vi "Display Error.vi"(8 "error in (no error)":errorcluster, 10 "Error message":string, 11 "Monitor-Pulse in":refnum<class "Monitor-Pulse.lvclass">) -> (0 "error out":errorcluster, 3 "Monitor-Pulse out":refnum<class "Monitor-Pulse.lvclass">)   [LabVIEW 2016, in "Monitor-Pulse.lvclass"]
uses:
  Monitor-Pulse.lvclass
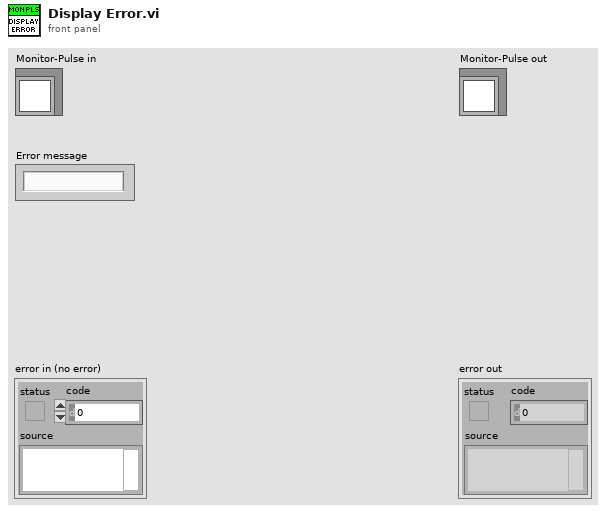
[diagram p1: front panel]
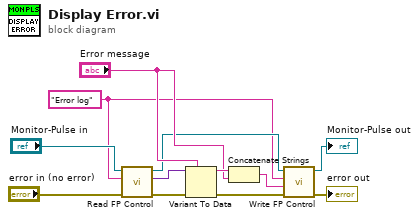
[diagram p0: block diagram]
diagram:
  w6 = "Error log" ("Control Name")
  n1 = call-dynamic "Read FP Control.vi"("error in (no error)"="error in (no error)", "Control Name"=w6, "Measure Object in"="Monitor-Pulse in") -> ("error out"=w10:errorcluster, "Control Value"=w11:variant, "Measure Object out"=w7:refnum<class "Monitor-Pulse.lvclass">)  [unwired: 5 in, 1 out]
  n2 = Variant To Data(error in=w10, type="Error message", Variant=w11) -> (data=w9:string, error out=w4:errorcluster)
  n3 = Concatenate Strings(w9, "Error message") -> (w5:string)
  n4 = call-dynamic "Write FP Control.vi"("error in (no error)"=w4, "Control Value"=w5, "Control Name"=w6, "Measure Object in"=w7) -> ("error out"=→"error out":errorcluster, "Measure Object out"=→"Monitor-Pulse out":refnum<class "Monitor-Pulse.lvclass">)  [unwired: 6 in]
